vi "Begin.vi"(11 "Image Size":T1=enum."320x240") -> (0 "error out":errorcluster)   [LabVIEW 2012]
doc: "Called before other user functions, this VI is expected to open initial I/O refnums, load in file data, and do all program initialization. Notice that the <B>error out</B> terminal is simply used for data flow. Wiring it to other structures or subVIs ensures that this VI runs first."
uses:
  <vilib>/Rock Robotics/WPI/Camera/WPI_CameraImageSize.ctl
  <vilib>/Rock Robotics/WPI/Joystick/WPI_JoystickDeviceEnum.ctl
  <vilib>/Rock Robotics/WPI/Camera/WPI_CameraWhite Balance Values.ctl
  <vilib>/Rock Robotics/WPI/Camera/WPI_CameraExposure Values.ctl
  <vilib>/Rock Robotics/WPI/Camera/WPI_CameraFrameRate.ctl
  <vilib>/Rock Robotics/SystemInterfaces/Typedef/FPGA_TypedefDigitalModule.ctl
  <vilib>/Rock Robotics/SystemInterfaces/DIO/FPGA_DIOPWMChannel.ctl
  <vilib>/Rock Robotics/SystemInterfaces/DIO/FPGA_DIOChannel.ctl
  <vilib>/Rock Robotics/WPI/CAN/Jaguar/SubVIs/WPI_CANJaguar_SpeedReference.ctl
  <vilib>/Rock Robotics/WPI/CAN/Jaguar/SubVIs/WPI_CANJaguar_ControlMode.ctl
  <vilib>/Rock Robotics/WPI/CAN/Jaguar/SubVIs/WPI_CANJaguar_PositionReference.ctl
  <vilib>/Rock Robotics/SystemInterfaces/DIO/FPGA_DIORelayChannel.ctl
  <vilib>/Rock Robotics/WPI/Relay/WPI_RelayDirection.ctl
  <vilib>/Rock Robotics/WPI/MotorControl/WPI_MotorControlOpenCANJaguar.vi
  <vilib>/Rock Robotics/WPI/MotorControl/WPI_MotorControlOpen Victor.vi
  <vilib>/Rock Robotics/WPI/RobotDrive/WPI_RobotDriveOpen4MotorWithCANJaguar.vi
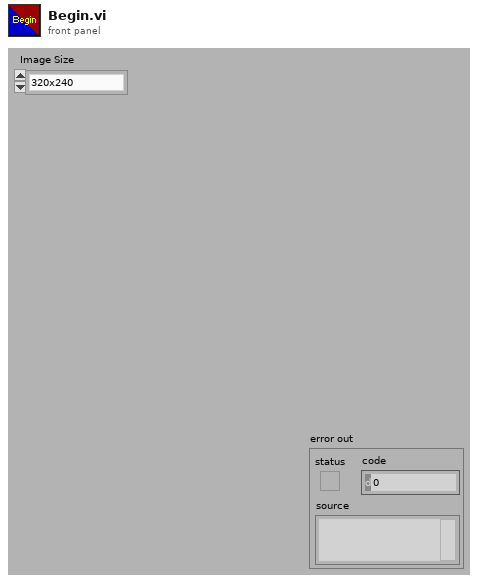
[diagram p1: front panel]
types:
  T1 = typedef "WPI_CameraImageSize.ctl" = enum16{"640x480", "320x240", "160x120"}
  T2 = typedef "WPI_CANJaguar_SpeedReference.ctl" = u8
  T3 = typedef "WPI_CANJaguar_ControlMode.ctl" = enum8{"Percent VBus", "Current", "Speed", "Position", "Voltage"}
  T4 = typedef "WPI_RelayDirection.ctl" = enum16{"Both directions", "Forward only", "Reverse only"}
  T5 = typedef "FPGA_DIORelayChannel.ctl" = enum8{"Relay 1", "Relay 2", "Relay 3", "Relay 4", "Relay 5", "Relay 6", "Relay 7", "Relay 8", "Invalid"}
  T6 = typedef "FPGA_DIOChannel.ctl" = enum8{"DIO 1", "DIO 2", "DIO 3", "DIO 4", "DIO 5", "DIO 6", "DIO 7", "DIO 8", "DIO 9", "DIO 10", "DIO 11", "DIO 12", "DIO 13", "DIO 14", "Invalid"}
  T7 = typedef "WPI_CANJaguar_PositionReference.ctl" = u8
  T8 = typedef "FPGA_DIOPWMChannel.ctl" = enum8{"PWM 1", "PWM 2", "PWM 3", "PWM 4", "PWM 5", "PWM 6", "PWM 7", "PWM 8", "PWM 9", "PWM 10", "Invalid"}
  T9 = typedef "FPGA_TypedefDigitalModule.ctl" = enum16{"Digital Module 1", "Digital Module 2"}
  T10 = typedef "WPI_JoystickDeviceEnum.ctl" = enum16{"USB 1", "USB 2", "USB 3", "USB 4", "Kinect 1", "Kinect 2"}
  T11 = typedef "WPI_CameraFrameRate.ctl" = u32
  T12 = typedef "WPI_CameraExposure Values.ctl" = enum16{"Auto", "Flicker-free 50 Hz", "Flicker-free 60 Hz", "Hold current"}
  T13 = typedef "WPI_CameraWhite Balance Values.ctl" = enum16{"Auto", "Fixed indoor", "Fixed outdoor 1", "Fixed outdoor 2", "Fixed fluorescent 1", "Fixed fluorescent 2", "Hold current"}
  T14 = typedef "WPI_RobotDriveDevRef.ctl" = cluster{"DevStatus":errorcluster, "Motors[]":T15[], "Square Inputs":bool, "Max Output":dbl, "Isochronous":bool}
  T15 = typedef "WPI_MotorControlDeviceRef.ctl" = cluster{"DeviceStatus":errorcluster, "Type":enum16{"PWM", "CAN"}, "PWM":cluster{"Digital Module":T9, "PWM Channel":T8, "DeadBand":T16}, "CAN":cluster{"Device Number":u8, "Control Mode":T3, "Semaphore":T17, "Max Vout":dbl}, "Invert":bool, "TransformRef":T18, "InvTransformRef":T18}
  T16 = typedef "WPI_PWMDeadband.ctl" = cluster{"Name":string, "maxPositivePwm":i32, "minPositivePwm":i32, "centerPwm":i32, "maxNegativePwm":i32, "minNegativePwm":i32, "angularRange":u16}
  T17 = typedef "Semaphore RefNum" = refnum<k1>
  T18 = typedef "WPI_PWMTransform_ConPane.ctl" = refnum<vi>
  T19 = typedef "WPI_JoystickDevRef.ctl" = cluster{"Device":T10}
  T20 = typedef "WPI_CameraDevRef.ctl" = cluster{"Camera Address":string, "CameraStatus":errorcluster, "Acquire Image Notifier":refnum<notifier>}
  T21 = typedef "WPI_DigitalInputDevRef.ctl" = cluster{"DevStatus":errorcluster, "DIO Channel":T6, "Digital Module":T9}
  T22 = typedef "WPI_RelayDevRef.ctl" = cluster{"DevStatus":errorcluster, "Relay Channel":T5, "Digital Module":T9, "Relay Direction":T4}
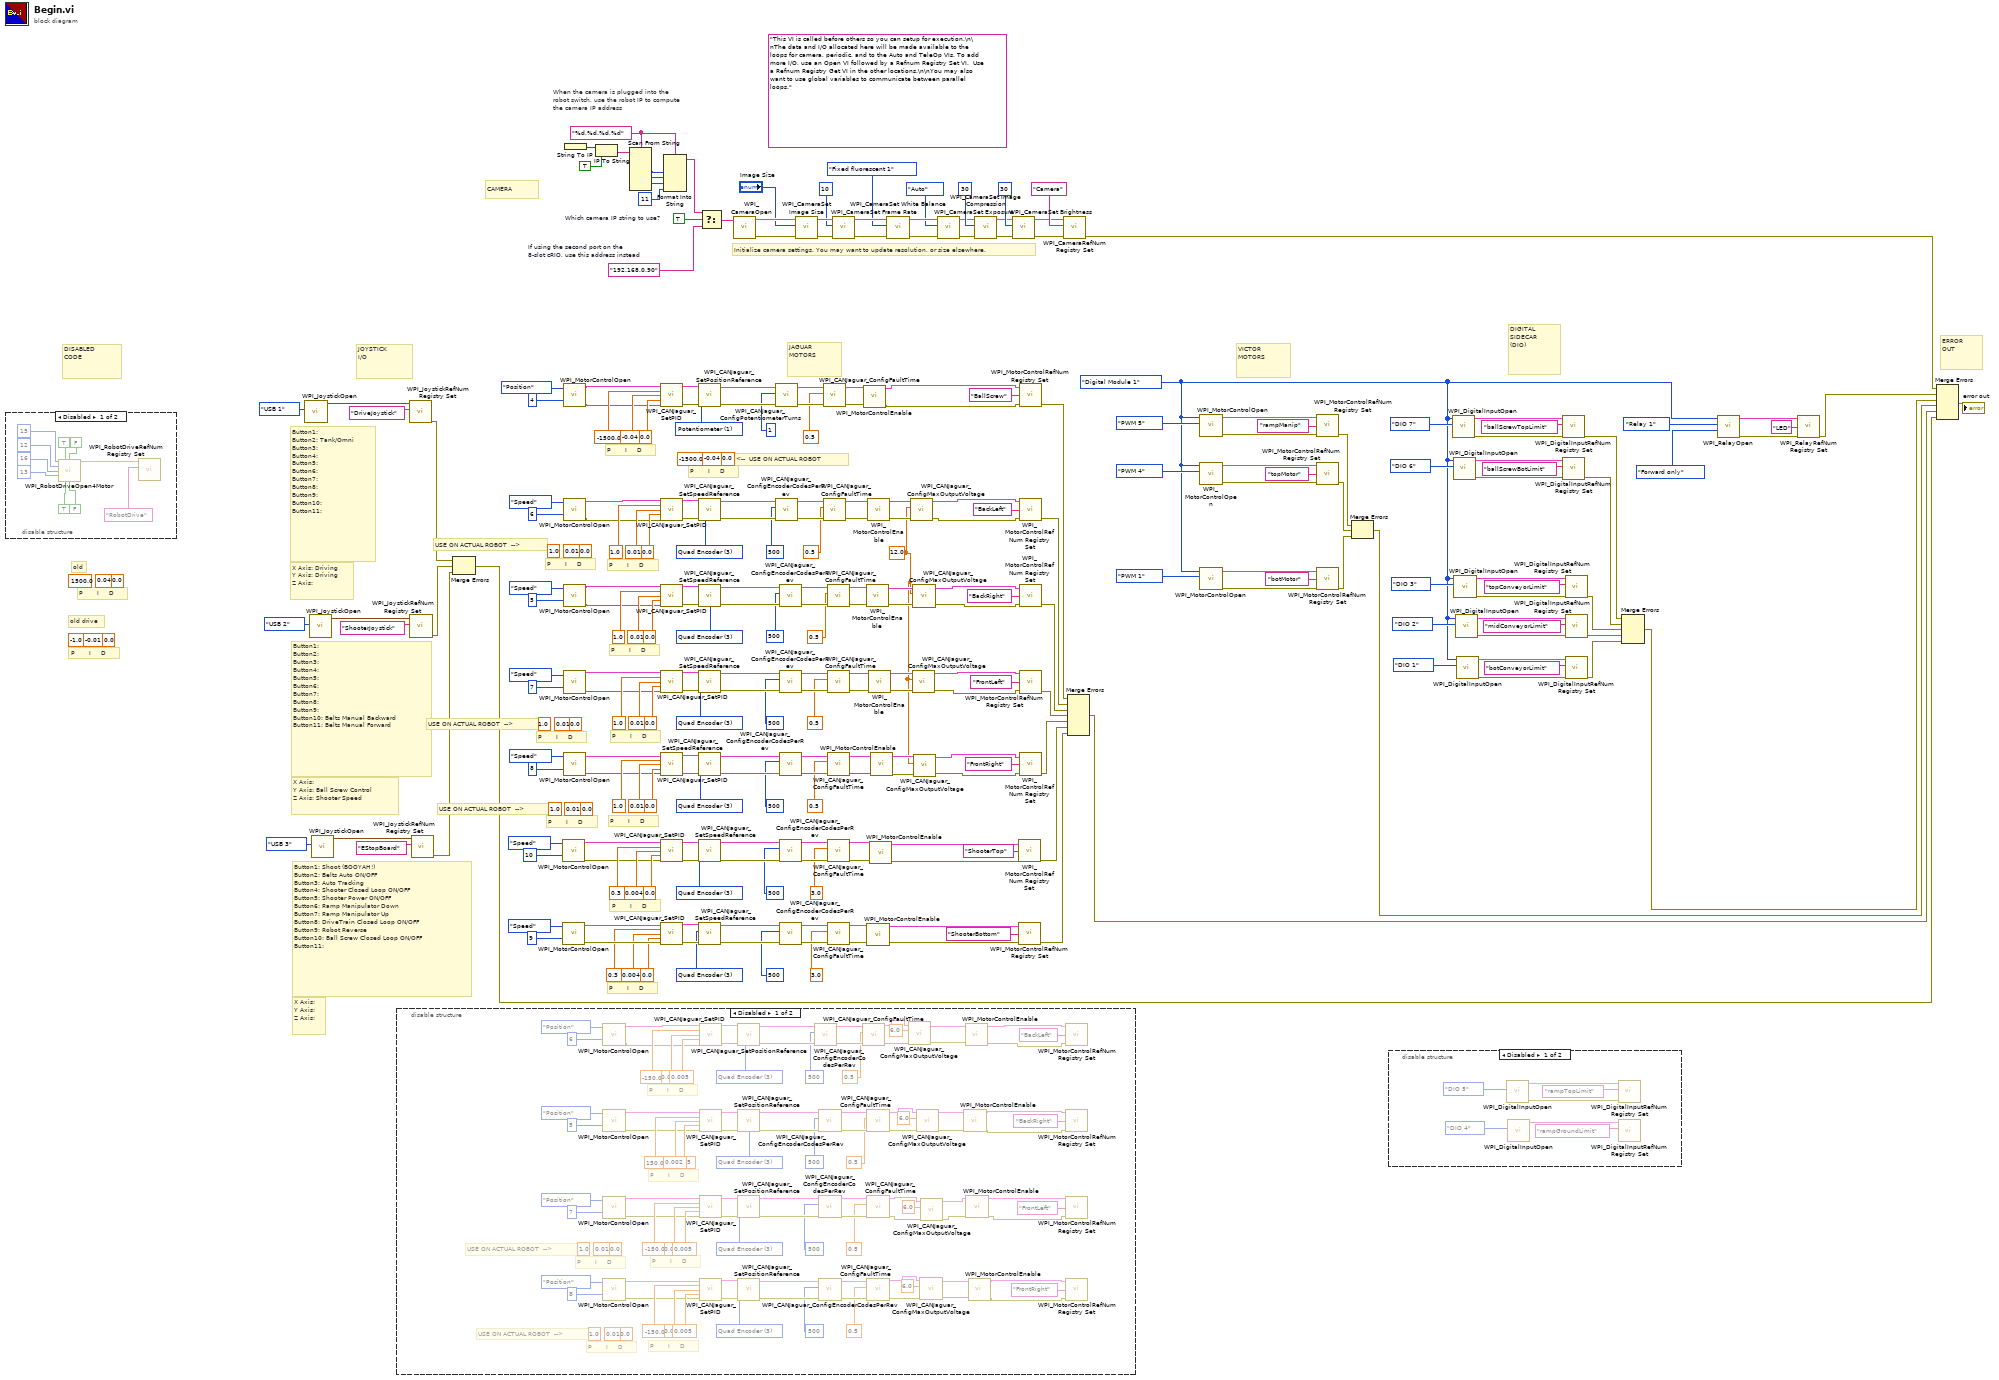
[diagram p0: block diagram]
diagram:
  (unwired) 0.0 ("D")
  (unwired) -0.01 ("I")
  (unwired) -1.0 ("P")
  (unwired) 0.0 ("D")
  (unwired) 0.04 ("I")
  (unwired) 1500.0 ("P")
  w4 = 12.0 ("Maximum Output Voltage")
  (unwired) 0.0 ("D")
  (unwired) 0.01 ("I")
  (unwired) 1.0 ("P")
  (unwired) 0.0 ("D")
  (unwired) 0.01 ("I")
  (unwired) 1.0 ("P")
  (unwired) 0.0 ("D")
  (unwired) 0.01 ("I")
  (unwired) 1.0 ("P")
  w37 = T2 3 items=["Encoder"=0, "Inv Encoder"=2, "Quad Encoder"=3, "None"=255] ("Speed Reference")
  w51 = T2 3 items=["Encoder"=0, "Inv Encoder"=2, "Quad Encoder"=3, "None"=255] ("Speed Reference")
  w65 = T2 3 items=["Encoder"=0, "Inv Encoder"=2, "Quad Encoder"=3, "None"=255] ("Speed Reference")
  w79 = T2 3 items=["Encoder"=0, "Inv Encoder"=2, "Quad Encoder"=3, "None"=255] ("Speed Reference")
  (unwired) 0.0 ("D")
  (unwired) -0.04 ("I")
  (unwired) -1500.0 ("P")
  w118 = T7 1 items=["Quad Encoder"=0, "Potentiometer"=1, "None"=255] ("Position Reference")
  w147 = T2 3 items=["Encoder"=0, "Inv Encoder"=2, "Quad Encoder"=3, "None"=255] ("Speed Reference")
  w161 = T2 3 items=["Encoder"=0, "Inv Encoder"=2, "Quad Encoder"=3, "None"=255] ("Speed Reference")
  w3 = FPGA_TypedefDigitalModule."Digital Module 1" ("Digital Module (Module 1)")
  w226 = TRUE  # Which camera IP string to use?
  w230 = "%d.%d.%d.%d" ("format string")
  (unwired) "This VI is called before others so you can setup for execution.\n\nThe data and I/O allocated here will be made available to the loops for camera, periodic, and to the Auto and TeleOp VIs. To add more I/O, use an Open VI followed by a Refnum Registry Set VI.  Use a Refnum Registry Get VI in the other locations.\n\nYou may also want to use global variables to communicate between parallel loops."
  w227 = "192.168.0.90"  # If using the second port on the 8-slot cRIO, use this address instead
  # "old drive"
  # "P       I     D"
  # "old"
  # "P       I     D"
  # "P       I     D"
  # "USE ON ACTUAL ROBOT  -->"
  # "P       I     D"
  # "USE ON ACTUAL ROBOT  -->"
  # "USE ON ACTUAL ROBOT  -->"
  # "P       I     D"
  # "P       I     D"
  # "P       I     D"
  # "P       I     D"
  # "P       I     D"
  # "<--  USE ON ACTUAL ROBOT"
  # "P       I     D"
  # "P       I     D"
  # "P       I     D"
  # "P       I     D"
  # "DIGITAL\nSIDECAR\n(DIO)"
  # "VICTOR\nMOTORS"
  # "X Axis:\nY Axis: \nZ Axis:"
  # "Button1: Shoot (BOOYAH!)\nButton2: Belts Auto ON/OFF\nButton3: Auto Tracking\nButton4: Shooter Closed Loop ON/OFF\nButton5: Shooter Power ON/OFF\nButton6: Ramp Manipulator Down\nButton7: Ramp Manipulator Up\nButton8: DriveTrain Closed Loop ON/OFF\nButton9: Robot Reverse\nButton10: Ball Screw Closed Loop ON/OFF\nButton11:"
  # "X Axis: \nY Axis: Ball Screw Control\nZ Axis: Shooter Speed"
  # "Button1:\nButton2: \nButton3:\nButton4:\nButton5:\nButton6:\nButton7:\nButton8:\nButton9:\nButton10: Belts Manual Backward\nButton11: Belts Manual Forward"
  # "X Axis: Driving\nY Axis: Driving\nZ Axis:"
  # "Button1:\nButton2: Tank/Omni\nButton3:\nButton4:\nButton5:\nButton6:\nButton7:\nButton8:\nButton9:\nButton10:\nButton11:"
  # "ERROR\nOUT"
  # "DISABLED\nCODE"
  # "CAMERA"
  # "JAGUAR\nMOTORS"
  # "JOYSTICK\nI/O"
  # "When the camera is plugged into the\nrobot switch, use the robot IP to compute\nthe camera IP address"
  # "Initialize camera settings. You may want to update resolution, or size elsewhere."
  n1 = disable-structure shown="Disabled" {
    frame Disabled {
      n2 = call-poly <vilib>:"WPI_RobotDriveOpen4Motor.vi"("Rear Left Motor"=u8 15, "Rear Left Motor Inverted"=TRUE, "Rear Right Motor Inverted"=FALSE, "Rear Right Motor"=u8 12, "Front Left Motor"=u8 16, "Front Right Motor"=u8 13, "Front Left Motor Inverted"=TRUE, "Front Right Motor Inverted"=FALSE) -> ("RobotDriveDevRef"=w263:T14)  [unwired: 6 in, 1 out]
      n3 = call <vilib>:"WPI_RobotDriveRefNum Registry Set.vi"("refnum name"="RobotDrive", "RobotDriveDevRef"=w263) -> ()  [unwired: 8 in, 2 out]
    }
    frame Enabled {
    }
  }
  n4 = call <vilib>:"WPI_JoystickOpen.vi"("JoystickDevice"=WPI_JoystickDeviceEnum."USB 1") -> ("JoystickDevRef"=w260:T19)  [unwired: 10 out]
  n5 = call <vilib>:"WPI_JoystickOpen.vi"("JoystickDevice"=WPI_JoystickDeviceEnum."USB 2") -> ("JoystickDevRef"=w211:T19)  [unwired: 10 out]
  n6 = call <vilib>:"WPI_JoystickOpen.vi"("JoystickDevice"=WPI_JoystickDeviceEnum."USB 3") -> ("JoystickDevRef"=w205:T19)  [unwired: 10 out]
  n7 = disable-structure shown="Disabled" {
    frame Disabled {
      (unwired) 0.0 ("D")
      (unwired) 0.01 ("I")
      (unwired) 1.0 ("P")
      (unwired) 0.0 ("D")
      (unwired) 0.01 ("I")
      (unwired) 1.0 ("P")
      w308 = T2 3 items=["Encoder"=0, "Inv Encoder"=2, "Quad Encoder"=3, "None"=255] ("Speed Reference")
      w322 = T2 3 items=["Encoder"=0, "Inv Encoder"=2, "Quad Encoder"=3, "None"=255] ("Speed Reference")
      w336 = T2 3 items=["Encoder"=0, "Inv Encoder"=2, "Quad Encoder"=3, "None"=255] ("Speed Reference")
      w350 = T2 3 items=["Encoder"=0, "Inv Encoder"=2, "Quad Encoder"=3, "None"=255] ("Speed Reference")
      # "P       I     D"
      # "USE ON ACTUAL ROBOT  -->"
      # "P       I     D"
      # "USE ON ACTUAL ROBOT  -->"
      # "P       I     D"
      # "P       I     D"
      # "P       I     D"
      # "P       I     D"
      n8 = call-poly <vilib>:"WPI_MotorControlOpen.vi"("Device Number"=u8 6, "Control Mode"=WPI_CANJaguar_ControlMode."Position") -> ("error out"=w300:errorcluster, "MotorControlDeviceRef"=w301:T15)  [unwired: 8 in]
      n9 = call-poly <vilib>:"WPI_MotorControlOpen.vi"("Device Number"=u8 5, "Control Mode"=WPI_CANJaguar_ControlMode."Position") -> ("error out"=w314:errorcluster, "MotorControlDeviceRef"=w315:T15)  [unwired: 8 in]
      n10 = call-poly <vilib>:"WPI_MotorControlOpen.vi"("Device Number"=u8 7, "Control Mode"=WPI_CANJaguar_ControlMode."Position") -> ("error out"=w328:errorcluster, "MotorControlDeviceRef"=w329:T15)  [unwired: 8 in]
      n11 = call-poly <vilib>:"WPI_MotorControlOpen.vi"("Device Number"=u8 8, "Control Mode"=WPI_CANJaguar_ControlMode."Position") -> ("error out"=w342:errorcluster, "MotorControlDeviceRef"=w343:T15)  [unwired: 8 in]
      n12 = call <vilib>:"WPI_CANJaguar_SetPID.vi"("CAN Jaguar Ref"=w301, "P"=-150.0, "I"=-0.002, "D"=0.005, "error in (no error)"=w300) -> ("CAN Jaguar Ref Out"=w309:T15, "error out"=w310:errorcluster)  [unwired: 9 in]
      n13 = call <vilib>:"WPI_CANJaguar_SetPID.vi"("CAN Jaguar Ref"=w315, "P"=150.0, "I"=0.002, "D"=0.005, "error in (no error)"=w314) -> ("CAN Jaguar Ref Out"=w323:T15, "error out"=w324:errorcluster)  [unwired: 9 in]
      n14 = call <vilib>:"WPI_CANJaguar_SetPID.vi"("CAN Jaguar Ref"=w329, "P"=-150.0, "I"=-0.002, "D"=0.005, "error in (no error)"=w328) -> ("CAN Jaguar Ref Out"=w337:T15, "error out"=w338:errorcluster)  [unwired: 9 in]
      n15 = call <vilib>:"WPI_CANJaguar_SetPID.vi"("CAN Jaguar Ref"=w343, "P"=-150.0, "I"=-0.002, "D"=0.005, "error in (no error)"=w342) -> ("CAN Jaguar Ref Out"=w351:T15, "error out"=w352:errorcluster)  [unwired: 9 in]
      n16 = call <vilib>:"WPI_CANJaguar_SetPositionReference.vi"("error in (no error)"=w310, "Position Reference"=w308, "CAN Jaguar Ref"=w309) -> ("error out"=w307:errorcluster, "CAN Jaguar Ref Out"=w306:T15)  [unwired: 7 in]
      n17 = call <vilib>:"WPI_CANJaguar_SetPositionReference.vi"("error in (no error)"=w324, "Position Reference"=w322, "CAN Jaguar Ref"=w323) -> ("error out"=w321:errorcluster, "CAN Jaguar Ref Out"=w320:T15)  [unwired: 7 in]
      n18 = call <vilib>:"WPI_CANJaguar_SetPositionReference.vi"("error in (no error)"=w338, "Position Reference"=w336, "CAN Jaguar Ref"=w337) -> ("error out"=w335:errorcluster, "CAN Jaguar Ref Out"=w334:T15)  [unwired: 7 in]
      n19 = call <vilib>:"WPI_CANJaguar_SetPositionReference.vi"("error in (no error)"=w352, "Position Reference"=w350, "CAN Jaguar Ref"=w351) -> ("error out"=w349:errorcluster, "CAN Jaguar Ref Out"=w348:T15)  [unwired: 7 in]
      n20 = call <vilib>:"WPI_CANJaguar_ConfigEncoderCodesPerRev.vi"("error in (no error)"=w307, "Encoder Codes Per Rev"=u16 500, "CAN Jaguar Ref"=w306) -> ("error out"=w304:errorcluster, "CAN Jaguar Ref Out"=w303:T15)  [unwired: 7 in]
      n21 = call <vilib>:"WPI_CANJaguar_ConfigEncoderCodesPerRev.vi"("error in (no error)"=w321, "Encoder Codes Per Rev"=u16 500, "CAN Jaguar Ref"=w320) -> ("error out"=w318:errorcluster, "CAN Jaguar Ref Out"=w317:T15)  [unwired: 7 in]
      n22 = call <vilib>:"WPI_CANJaguar_ConfigEncoderCodesPerRev.vi"("error in (no error)"=w335, "Encoder Codes Per Rev"=u16 500, "CAN Jaguar Ref"=w334) -> ("error out"=w332:errorcluster, "CAN Jaguar Ref Out"=w331:T15)  [unwired: 7 in]
      n23 = call <vilib>:"WPI_CANJaguar_ConfigEncoderCodesPerRev.vi"("error in (no error)"=w349, "Encoder Codes Per Rev"=u16 500, "CAN Jaguar Ref"=w348) -> ("error out"=w346:errorcluster, "CAN Jaguar Ref Out"=w345:T15)  [unwired: 7 in]
      n24 = call <vilib>:"WPI_CANJaguar_ConfigFaultTime.vi"("error in (no error)"=w304, "Fault Time (s)"=0.5, "CAN Jaguar Ref"=w303) -> ("error out"=w275:errorcluster, "CAN Jaguar Ref Out"=w272:T15)  [unwired: 7 in]
      n25 = call <vilib>:"WPI_CANJaguar_ConfigFaultTime.vi"("error in (no error)"=w318, "Fault Time (s)"=0.5, "CAN Jaguar Ref"=w317) -> ("error out"=w279:errorcluster, "CAN Jaguar Ref Out"=w276:T15)  [unwired: 7 in]
      n26 = call <vilib>:"WPI_CANJaguar_ConfigFaultTime.vi"("error in (no error)"=w332, "Fault Time (s)"=0.5, "CAN Jaguar Ref"=w331) -> ("error out"=w283:errorcluster, "CAN Jaguar Ref Out"=w280:T15)  [unwired: 7 in]
      n27 = call <vilib>:"WPI_CANJaguar_ConfigFaultTime.vi"("error in (no error)"=w346, "Fault Time (s)"=0.5, "CAN Jaguar Ref"=w345) -> ("error out"=w287:errorcluster, "CAN Jaguar Ref Out"=w284:T15)  [unwired: 7 in]
      n28 = call <vilib>:"WPI_CANJaguar_ConfigMaxOutputVoltage.vi"("error in (no error)"=w275, "Maximum Output Voltage"=6.0, "CAN Jaguar Ref"=w272) -> ("error out"=w274:errorcluster, "CAN Jaguar Ref Out"=w273:T15)  [unwired: 7 in]
      n29 = call <vilib>:"WPI_CANJaguar_ConfigMaxOutputVoltage.vi"("error in (no error)"=w279, "Maximum Output Voltage"=6.0, "CAN Jaguar Ref"=w276) -> ("error out"=w278:errorcluster, "CAN Jaguar Ref Out"=w277:T15)  [unwired: 7 in]
      n30 = call <vilib>:"WPI_CANJaguar_ConfigMaxOutputVoltage.vi"("error in (no error)"=w287, "Maximum Output Voltage"=6.0, "CAN Jaguar Ref"=w284) -> ("error out"=w286:errorcluster, "CAN Jaguar Ref Out"=w285:T15)  [unwired: 7 in]
      n31 = call <vilib>:"WPI_CANJaguar_ConfigMaxOutputVoltage.vi"("error in (no error)"=w283, "Maximum Output Voltage"=6.0, "CAN Jaguar Ref"=w280) -> ("error out"=w282:errorcluster, "CAN Jaguar Ref Out"=w281:T15)  [unwired: 7 in]
      n32 = call <vilib>:"WPI_MotorControlEnable.vi"("error in (no error)"=w278, "CAN Jaguar Ref"=w277) -> ("error out"=w296:errorcluster, "CAN Jaguar Ref Out"=w297:T15)  [unwired: 8 in]
      n33 = call <vilib>:"WPI_MotorControlEnable.vi"("error in (no error)"=w274, "CAN Jaguar Ref"=w273) -> ("error out"=w298:errorcluster, "CAN Jaguar Ref Out"=w299:T15)  [unwired: 8 in]
      n34 = call <vilib>:"WPI_MotorControlEnable.vi"("error in (no error)"=w282, "CAN Jaguar Ref"=w281) -> ("error out"=w295:errorcluster, "CAN Jaguar Ref Out"=w294:T15)  [unwired: 8 in]
      n35 = call <vilib>:"WPI_MotorControlEnable.vi"("error in (no error)"=w286, "CAN Jaguar Ref"=w285) -> ("error out"=w292:errorcluster, "CAN Jaguar Ref Out"=w293:T15)  [unwired: 8 in]
      n36 = call <vilib>:"WPI_MotorControlRefNum Registry Set.vi"("error in (no error)"=w298, "refnum name"="BackLeft", "MotorControlDevRef"=w299) -> ()  [unwired: 7 in, 2 out]
      n37 = call <vilib>:"WPI_MotorControlRefNum Registry Set.vi"("error in (no error)"=w296, "refnum name"="BackRight", "MotorControlDevRef"=w297) -> ()  [unwired: 7 in, 2 out]
      n38 = call <vilib>:"WPI_MotorControlRefNum Registry Set.vi"("error in (no error)"=w295, "refnum name"="FrontLeft", "MotorControlDevRef"=w294) -> ()  [unwired: 7 in, 2 out]
      n39 = call <vilib>:"WPI_MotorControlRefNum Registry Set.vi"("error in (no error)"=w292, "refnum name"="FrontRight", "MotorControlDevRef"=w293) -> ()  [unwired: 7 in, 2 out]
    }
    frame Enabled {
    }
  }
  n40 = call <vilib>:"WPI_JoystickRefNum Registry Set.vi"("refnum name"="DriveJoystick", "JoystickDevRef"=w260) -> ("error out"=w207:errorcluster)  [unwired: 1 in, 8 out]
  n41 = call <vilib>:"WPI_JoystickRefNum Registry Set.vi"("refnum name"="ShooterJoystick", "JoystickDevRef"=w211) -> ("error out"=w206:errorcluster)  [unwired: 1 in, 8 out]
  n42 = call <vilib>:"WPI_JoystickRefNum Registry Set.vi"("refnum name"="EStopBoard", "JoystickDevRef"=w205) -> ("error out"=w202:errorcluster)  [unwired: 1 in, 8 out]
  n43 = Merge Errors(w207, w206, w202) -> (w208:errorcluster)
  n44 = call-poly <vilib>:"WPI_MotorControlOpen.vi"("Device Number"=u8 10, "Control Mode"=WPI_CANJaguar_ControlMode."Speed") -> ("error out"=w137:errorcluster, "MotorControlDeviceRef"=w138:T15)  [unwired: 8 in]
  n45 = call-poly <vilib>:"WPI_MotorControlOpen.vi"("Device Number"=u8 9, "Control Mode"=WPI_CANJaguar_ControlMode."Speed") -> ("error out"=w167:errorcluster, "MotorControlDeviceRef"=w168:T15)  [unwired: 8 in]
  n46 = call-poly <vilib>:"WPI_MotorControlOpen.vi"("Device Number"=u8 4, "Control Mode"=WPI_CANJaguar_ControlMode."Position") -> ("error out"=w119:errorcluster, "MotorControlDeviceRef"=w120:T15)  [unwired: 8 in]
  n47 = call-poly <vilib>:"WPI_MotorControlOpen.vi"("Device Number"=u8 6, "Control Mode"=WPI_CANJaguar_ControlMode."Speed") -> ("error out"=w29:errorcluster, "MotorControlDeviceRef"=w30:T15)  [unwired: 8 in]
  n48 = call-poly <vilib>:"WPI_MotorControlOpen.vi"("Device Number"=u8 5, "Control Mode"=WPI_CANJaguar_ControlMode."Speed") -> ("error out"=w43:errorcluster, "MotorControlDeviceRef"=w44:T15)  [unwired: 8 in]
  n49 = call-poly <vilib>:"WPI_MotorControlOpen.vi"("Device Number"=u8 7, "Control Mode"=WPI_CANJaguar_ControlMode."Speed") -> ("error out"=w57:errorcluster, "MotorControlDeviceRef"=w58:T15)  [unwired: 8 in]
  n50 = call-poly <vilib>:"WPI_MotorControlOpen.vi"("Device Number"=u8 8, "Control Mode"=WPI_CANJaguar_ControlMode."Speed") -> ("error out"=w71:errorcluster, "MotorControlDeviceRef"=w72:T15)  [unwired: 8 in]
  n51 = String To IP() -> (0:w237:u32)  [unwired: 1 in]
  n52 = IP To String(1:TRUE ("dot notation? (F)"), 2:w237) -> (0:w235:string)
  n53 = Scan From String(format string=w230, input string=w235) -> (output 1=w234:i32, output 2=w233:i32, output 3=w232:i32)  [unwired: 7 in, 3 out]
  n54 = call <vilib>:"WPI_CANJaguar_SetPID.vi"("CAN Jaguar Ref"=w120, "P"=-1500.0, "I"=-0.04, "D"=0.0, "error in (no error)"=w119) -> ("CAN Jaguar Ref Out"=w126:T15, "error out"=w127:errorcluster)  [unwired: 9 in]
  n55 = call <vilib>:"WPI_CANJaguar_SetPID.vi"("CAN Jaguar Ref"=w30, "P"=1.0, "I"=0.01, "D"=0.0, "error in (no error)"=w29) -> ("CAN Jaguar Ref Out"=w38:T15, "error out"=w39:errorcluster)  [unwired: 9 in]
  n56 = call <vilib>:"WPI_CANJaguar_SetPID.vi"("CAN Jaguar Ref"=w44, "P"=1.0, "I"=0.01, "D"=0.0, "error in (no error)"=w43) -> ("CAN Jaguar Ref Out"=w52:T15, "error out"=w53:errorcluster)  [unwired: 9 in]
  n57 = call <vilib>:"WPI_CANJaguar_SetPID.vi"("CAN Jaguar Ref"=w58, "P"=1.0, "I"=0.01, "D"=0.0, "error in (no error)"=w57) -> ("CAN Jaguar Ref Out"=w66:T15, "error out"=w67:errorcluster)  [unwired: 9 in]
  n58 = call <vilib>:"WPI_CANJaguar_SetPID.vi"("CAN Jaguar Ref"=w72, "P"=1.0, "I"=0.01, "D"=0.0, "error in (no error)"=w71) -> ("CAN Jaguar Ref Out"=w80:T15, "error out"=w81:errorcluster)  [unwired: 9 in]
  n59 = call <vilib>:"WPI_CANJaguar_SetPID.vi"("CAN Jaguar Ref"=w138, "P"=0.3, "I"=0.004, "D"=0.0, "error in (no error)"=w137) -> ("CAN Jaguar Ref Out"=w148:T15, "error out"=w149:errorcluster)  [unwired: 9 in]
  n60 = call <vilib>:"WPI_CANJaguar_SetPID.vi"("CAN Jaguar Ref"=w168, "P"=0.3, "I"=0.004, "D"=0.0, "error in (no error)"=w167) -> ("CAN Jaguar Ref Out"=w162:T15, "error out"=w163:errorcluster)  [unwired: 9 in]
  n61 = Format Into String(format string=w230, w234, w233, w232, 11 ("Compression")) -> (resulting string=w228:string)  [unwired: 2 in, 1 out]
  n62 = call <vilib>:"WPI_CANJaguar_SetPositionReference.vi"("error in (no error)"=w127, "Position Reference"=w118, "CAN Jaguar Ref"=w126) -> ("error out"=w125:errorcluster, "CAN Jaguar Ref Out"=w124:T15)  [unwired: 7 in]
  n63 = call <vilib>:"WPI_CANJaguar_SetSpeedReference.vi"("error in (no error)"=w39, "Speed Reference"=w37, "CAN Jaguar Ref"=w38) -> ("error out"=w36:errorcluster, "CAN Jaguar Ref Out"=w35:T15)  [unwired: 7 in]
  n64 = call <vilib>:"WPI_CANJaguar_SetSpeedReference.vi"("error in (no error)"=w53, "Speed Reference"=w51, "CAN Jaguar Ref"=w52) -> ("error out"=w50:errorcluster, "CAN Jaguar Ref Out"=w49:T15)  [unwired: 7 in]
  n65 = call <vilib>:"WPI_CANJaguar_SetSpeedReference.vi"("error in (no error)"=w67, "Speed Reference"=w65, "CAN Jaguar Ref"=w66) -> ("error out"=w64:errorcluster, "CAN Jaguar Ref Out"=w63:T15)  [unwired: 7 in]
  n66 = call <vilib>:"WPI_CANJaguar_SetSpeedReference.vi"("error in (no error)"=w81, "Speed Reference"=w79, "CAN Jaguar Ref"=w80) -> ("error out"=w78:errorcluster, "CAN Jaguar Ref Out"=w77:T15)  [unwired: 7 in]
  n67 = call <vilib>:"WPI_CANJaguar_SetSpeedReference.vi"("error in (no error)"=w149, "Speed Reference"=w147, "CAN Jaguar Ref"=w148) -> ("error out"=w146:errorcluster, "CAN Jaguar Ref Out"=w145:T15)  [unwired: 7 in]
  n68 = call <vilib>:"WPI_CANJaguar_SetSpeedReference.vi"("error in (no error)"=w163, "Speed Reference"=w161, "CAN Jaguar Ref"=w162) -> ("error out"=w160:errorcluster, "CAN Jaguar Ref Out"=w159:T15)  [unwired: 7 in]
  n69 = Select(t=w228, s=w226, f=w227) -> (s? t:f=w229:string)
  n70 = call <vilib>:"WPI_CameraOpen.vi"("Camera Address"=w229) -> ("error out"=w250:errorcluster, "CameraDevRef"=w251:T20)  [unwired: 1 in, 8 out]
  n71 = call <vilib>:"WPI_CANJaguar_ConfigPotentiometerTurns.vi"("error in (no error)"=w125, "Potentiometer Turns"=u16 1, "CAN Jaguar Ref"=w124) -> ("error out"=w123:errorcluster, "CAN Jaguar Ref Out"=w122:T15)  [unwired: 7 in]
  n72 = call <vilib>:"WPI_CANJaguar_ConfigEncoderCodesPerRev.vi"("error in (no error)"=w36, "Encoder Codes Per Rev"=u16 500, "CAN Jaguar Ref"=w35) -> ("error out"=w33:errorcluster, "CAN Jaguar Ref Out"=w32:T15)  [unwired: 7 in]
  n73 = call <vilib>:"WPI_CANJaguar_ConfigEncoderCodesPerRev.vi"("error in (no error)"=w50, "Encoder Codes Per Rev"=u16 500, "CAN Jaguar Ref"=w49) -> ("error out"=w47:errorcluster, "CAN Jaguar Ref Out"=w46:T15)  [unwired: 7 in]
  n74 = call <vilib>:"WPI_CANJaguar_ConfigEncoderCodesPerRev.vi"("error in (no error)"=w64, "Encoder Codes Per Rev"=u16 500, "CAN Jaguar Ref"=w63) -> ("error out"=w61:errorcluster, "CAN Jaguar Ref Out"=w60:T15)  [unwired: 7 in]
  n75 = call <vilib>:"WPI_CANJaguar_ConfigEncoderCodesPerRev.vi"("error in (no error)"=w78, "Encoder Codes Per Rev"=u16 500, "CAN Jaguar Ref"=w77) -> ("error out"=w75:errorcluster, "CAN Jaguar Ref Out"=w74:T15)  [unwired: 7 in]
  n76 = call <vilib>:"WPI_CANJaguar_ConfigEncoderCodesPerRev.vi"("error in (no error)"=w146, "Encoder Codes Per Rev"=u16 500, "CAN Jaguar Ref"=w145) -> ("error out"=w143:errorcluster, "CAN Jaguar Ref Out"=w142:T15)  [unwired: 7 in]
  n77 = call <vilib>:"WPI_CANJaguar_ConfigEncoderCodesPerRev.vi"("error in (no error)"=w160, "Encoder Codes Per Rev"=u16 500, "CAN Jaguar Ref"=w159) -> ("error out"=w157:errorcluster, "CAN Jaguar Ref Out"=w156:T15)  [unwired: 7 in]
  n78 = call <vilib>:"WPI_CameraSet Image Size.vi"("error in (no error)"=w250, "Image Size"="Image Size", "CameraDevRef"=w251) -> ("error out"=w249:errorcluster, "CameraDevRef Out"=w252:T20)  [unwired: 7 out]
  n79 = call <vilib>:"WPI_CANJaguar_ConfigFaultTime.vi"("error in (no error)"=w123, "Fault Time (s)"=0.5, "CAN Jaguar Ref"=w122) -> ("error out"=w107:errorcluster, "CAN Jaguar Ref Out"=w108:T15)  [unwired: 7 in]
  n80 = call <vilib>:"WPI_CANJaguar_ConfigFaultTime.vi"("error in (no error)"=w33, "Fault Time (s)"=0.5, "CAN Jaguar Ref"=w32) -> ("error out"=w28:errorcluster, "CAN Jaguar Ref Out"=w27:T15)  [unwired: 7 in]
  n81 = call <vilib>:"WPI_CANJaguar_ConfigFaultTime.vi"("error in (no error)"=w47, "Fault Time (s)"=0.5, "CAN Jaguar Ref"=w46) -> ("error out"=w25:errorcluster, "CAN Jaguar Ref Out"=w26:T15)  [unwired: 7 in]
  n82 = call <vilib>:"WPI_CANJaguar_ConfigFaultTime.vi"("error in (no error)"=w61, "Fault Time (s)"=0.5, "CAN Jaguar Ref"=w60) -> ("error out"=w23:errorcluster, "CAN Jaguar Ref Out"=w24:T15)  [unwired: 7 in]
  n83 = call <vilib>:"WPI_CANJaguar_ConfigFaultTime.vi"("error in (no error)"=w75, "Fault Time (s)"=0.5, "CAN Jaguar Ref"=w74) -> ("error out"=w22:errorcluster, "CAN Jaguar Ref Out"=w21:T15)  [unwired: 7 in]
  n84 = call <vilib>:"WPI_CANJaguar_ConfigFaultTime.vi"("error in (no error)"=w143, "Fault Time (s)"=3.0, "CAN Jaguar Ref"=w142) -> ("error out"=w139:errorcluster, "CAN Jaguar Ref Out"=w140:T15)  [unwired: 7 in]
  n85 = call <vilib>:"WPI_CANJaguar_ConfigFaultTime.vi"("error in (no error)"=w157, "Fault Time (s)"=3.0, "CAN Jaguar Ref"=w156) -> ("error out"=w153:errorcluster, "CAN Jaguar Ref Out"=w154:T15)  [unwired: 7 in]
  n86 = call <vilib>:"WPI_CameraSet Frame Rate.vi"("error in (no error)"=w249, "Frame Rate (fps)"=T11 10, "CameraDevRef"=w252) -> ("error out"=w248:errorcluster, "CameraDevRef Out"=w254:T20)  [unwired: 7 out]
  n87 = call <vilib>:"WPI_MotorControlEnable.vi"("error in (no error)"=w107, "CAN Jaguar Ref"=w108) -> ("error out"=w106:errorcluster, "CAN Jaguar Ref Out"=w105:T15)  [unwired: 8 in]
  n88 = call <vilib>:"WPI_MotorControlEnable.vi"("error in (no error)"=w25, "CAN Jaguar Ref"=w26) -> ("error out"=w16:errorcluster, "CAN Jaguar Ref Out"=w15:T15)  [unwired: 8 in]
  n89 = call <vilib>:"WPI_MotorControlEnable.vi"("error in (no error)"=w153, "CAN Jaguar Ref"=w154) -> ("error out"=w169:errorcluster, "CAN Jaguar Ref Out"=w170:T15)  [unwired: 8 in]
  n90 = call <vilib>:"WPI_MotorControlEnable.vi"("error in (no error)"=w28, "CAN Jaguar Ref"=w27) -> ("error out"=w19:errorcluster, "CAN Jaguar Ref Out"=w20:T15)  [unwired: 8 in]
  n91 = call <vilib>:"WPI_MotorControlEnable.vi"("error in (no error)"=w23, "CAN Jaguar Ref"=w24) -> ("error out"=w11:errorcluster, "CAN Jaguar Ref Out"=w12:T15)  [unwired: 8 in]
  n92 = call <vilib>:"WPI_MotorControlEnable.vi"("error in (no error)"=w139, "CAN Jaguar Ref"=w140) -> ("error out"=w136:errorcluster, "CAN Jaguar Ref Out"=w135:T15)  [unwired: 8 in]
  n93 = call <vilib>:"WPI_MotorControlEnable.vi"("error in (no error)"=w22, "CAN Jaguar Ref"=w21) -> ("error out"=w5:errorcluster, "CAN Jaguar Ref Out"=w8:T15)  [unwired: 8 in]
  n94 = call <vilib>:"WPI_CameraSet White Balance.vi"("error in (no error)"=w248, "White Balance"=WPI_CameraWhite_Balance_Values."Fixed fluorescent 1", "CameraDevRef"=w254) -> ("error out"=w247:errorcluster, "CameraDevRef Out"=w253:T20)  [unwired: 7 out]
  n95 = call <vilib>:"WPI_CANJaguar_ConfigMaxOutputVoltage.vi"("error in (no error)"=w19, "Maximum Output Voltage"=w4, "CAN Jaguar Ref"=w20) -> ("error out"=w18:errorcluster, "CAN Jaguar Ref Out"=w17:T15)  [unwired: 7 in]
  n96 = call <vilib>:"WPI_CANJaguar_ConfigMaxOutputVoltage.vi"("error in (no error)"=w11, "Maximum Output Voltage"=w4, "CAN Jaguar Ref"=w12) -> ("error out"=w10:errorcluster, "CAN Jaguar Ref Out"=w9:T15)  [unwired: 7 in]
  n97 = call <vilib>:"WPI_CANJaguar_ConfigMaxOutputVoltage.vi"("error in (no error)"=w16, "Maximum Output Voltage"=w4, "CAN Jaguar Ref"=w15) -> ("error out"=w13:errorcluster, "CAN Jaguar Ref Out"=w14:T15)  [unwired: 7 in]
  n98 = call <vilib>:"WPI_CANJaguar_ConfigMaxOutputVoltage.vi"("error in (no error)"=w5, "Maximum Output Voltage"=w4, "CAN Jaguar Ref"=w8) -> ("error out"=w6:errorcluster, "CAN Jaguar Ref Out"=w7:T15)  [unwired: 7 in]
  n99 = call <vilib>:"WPI_CameraSet Exposure.vi"("error in (no error)"=w247, "Exposure"=WPI_CameraExposure_Values."Auto", "CameraDevRef"=w253) -> ("error out"=w246:errorcluster, "CameraDevRef Out"=w256:T20)  [unwired: 7 out]
  n100 = call <vilib>:"WPI_CameraSet Image Compression.vi"("error in (no error)"=w246, "Compression"=30, "CameraDevRef"=w256) -> ("error out"=w245:errorcluster, "CameraDevRef Out"=w255:T20)  [unwired: 7 out]
  n101 = call <vilib>:"WPI_CameraSet Brightness.vi"("error in (no error)"=w245, "Brightness"=30, "CameraDevRef"=w255) -> ("error out"=w243:errorcluster, "CameraDevRef Out"=w244:T20)  [unwired: 7 out]
  n102 = call <vilib>:"WPI_MotorControlRefNum Registry Set.vi"("error in (no error)"=w136, "refnum name"="ShooterTop", "MotorControlDevRef"=w135) -> ("error out"=w213:errorcluster)  [unwired: 7 in, 1 out]
  n103 = call <vilib>:"WPI_MotorControlRefNum Registry Set.vi"("error in (no error)"=w169, "refnum name"="ShooterBottom", "MotorControlDevRef"=w170) -> ("error out"=w212:errorcluster)  [unwired: 7 in, 1 out]
  n104 = call <vilib>:"WPI_MotorControlRefNum Registry Set.vi"("error in (no error)"=w106, "refnum name"="BallScrew", "MotorControlDevRef"=w105) -> ("error out"=w131:errorcluster)  [unwired: 7 in, 1 out]
  n105 = call <vilib>:"WPI_MotorControlRefNum Registry Set.vi"("error in (no error)"=w18, "refnum name"="BackLeft", "MotorControlDevRef"=w17) -> ("error out"=w224:errorcluster)  [unwired: 7 in, 1 out]
  n106 = call <vilib>:"WPI_MotorControlRefNum Registry Set.vi"("error in (no error)"=w13, "refnum name"="BackRight", "MotorControlDevRef"=w14) -> ("error out"=w223:errorcluster)  [unwired: 7 in, 1 out]
  n107 = call <vilib>:"WPI_MotorControlRefNum Registry Set.vi"("error in (no error)"=w10, "refnum name"="FrontLeft", "MotorControlDevRef"=w9) -> ("error out"=w222:errorcluster)  [unwired: 7 in, 1 out]
  n108 = call <vilib>:"WPI_MotorControlRefNum Registry Set.vi"("error in (no error)"=w6, "refnum name"="FrontRight", "MotorControlDevRef"=w7) -> ("error out"=w221:errorcluster)  [unwired: 7 in, 1 out]
  n109 = call <vilib>:"WPI_CameraRefNum Registry Set.vi"("error in (no error)"=w243, "refnum name"="Camera", "CameraDevRef"=w244) -> ("error out"=w98:errorcluster)  [unwired: 8 out]
  n110 = Merge Errors(w131, w224, w223, w222, w221, w213, w212) -> (w220:errorcluster)
  n111 = call-poly <vilib>:"WPI_MotorControlOpen.vi"("PWM Channel"=FPGA_DIOPWMChannel."PWM 5", "Digital Module (Module 1)"=w3) -> ("error out"=w175:errorcluster, "MotorControlDeviceRef"=w174:T15)  [unwired: 8 in]
  n112 = call-poly <vilib>:"WPI_MotorControlOpen.vi"("PWM Channel"=FPGA_DIOPWMChannel."PWM 4", "Digital Module (Module 1)"=w3) -> ("error out"=w201:errorcluster, "MotorControlDeviceRef"=w200:T15)  [unwired: 8 in]
  n113 = call-poly <vilib>:"WPI_MotorControlOpen.vi"("PWM Channel"=FPGA_DIOPWMChannel."PWM 1", "Digital Module (Module 1)"=w3) -> ("error out"=w198:errorcluster, "MotorControlDeviceRef"=w197:T15)  [unwired: 8 in]
  n114 = call <vilib>:"WPI_MotorControlRefNum Registry Set.vi"("error in (no error)"=w175, "refnum name"="rampManip", "MotorControlDevRef"=w174) -> ("error out"=w171:errorcluster)  [unwired: 7 in, 1 out]
  n115 = call <vilib>:"WPI_MotorControlRefNum Registry Set.vi"("error in (no error)"=w201, "refnum name"="topMotor", "MotorControlDevRef"=w200) -> ("error out"=w193:errorcluster)  [unwired: 7 in, 1 out]
  n116 = call <vilib>:"WPI_MotorControlRefNum Registry Set.vi"("error in (no error)"=w198, "refnum name"="botMotor", "MotorControlDevRef"=w197) -> ("error out"=w104:errorcluster)  [unwired: 7 in, 1 out]
  n117 = Merge Errors(w171, w193, w104) -> (w192:errorcluster)
  n118 = disable-structure shown="Disabled" {
    frame Disabled {
      n119 = call <vilib>:"WPI_DigitalInputOpen.vi"("DIO Channel"=FPGA_DIOChannel."DIO 5") -> ("error out"=w373:errorcluster, "DigitalInputDevRef"=w374:T21)  [unwired: 9 in]
      n120 = call <vilib>:"WPI_DigitalInputOpen.vi"("DIO Channel"=FPGA_DIOChannel."DIO 4") -> ("DigitalInputDevRef"=w368:T21)  [unwired: 9 in, 1 out]
      n121 = call <vilib>:"WPI_DigitalInputRefNum Registry Set.vi"("error in (no error)"=w373, "refnum name"="rampTopLimit", "DigitalInputDevRef"=w374) -> ()  [unwired: 7 in, 2 out]
      n122 = call <vilib>:"WPI_DigitalInputRefNum Registry Set.vi"("refnum name"="rampGroundLimit", "DigitalInputDevRef"=w368) -> ()  [unwired: 8 in, 2 out]
    }
    frame Enabled {
    }
  }
  n123 = call <vilib>:"WPI_DigitalInputOpen.vi"("DIO Channel"=FPGA_DIOChannel."DIO 7", "Digital Module (Module 1)"=w3) -> ("error out"=w116:errorcluster, "DigitalInputDevRef"=w113:T21)  [unwired: 8 in]
  n124 = call <vilib>:"WPI_DigitalInputOpen.vi"("DIO Channel"=FPGA_DIOChannel."DIO 6", "Digital Module (Module 1)"=w3) -> ("error out"=w112:errorcluster, "DigitalInputDevRef"=w109:T21)  [unwired: 8 in]
  n125 = call <vilib>:"WPI_DigitalInputOpen.vi"("DIO Channel"=FPGA_DIOChannel."DIO 3", "Digital Module (Module 1)"=w3) -> ("error out"=w190:errorcluster, "DigitalInputDevRef"=w191:T21)  [unwired: 8 in]
  n126 = call <vilib>:"WPI_DigitalInputOpen.vi"("DIO Channel"=FPGA_DIOChannel."DIO 2", "Digital Module (Module 1)"=w3) -> ("error out"=w187:errorcluster, "DigitalInputDevRef"=w184:T21)  [unwired: 8 in]
  n127 = call <vilib>:"WPI_DigitalInputOpen.vi"("DIO Channel"=FPGA_DIOChannel."DIO 1", "Digital Module (Module 1)"=w3) -> ("error out"=w183:errorcluster, "DigitalInputDevRef"=w180:T21)  [unwired: 8 in]
  n128 = call <vilib>:"WPI_DigitalInputRefNum Registry Set.vi"("error in (no error)"=w116, "refnum name"="ballScrewTopLimit", "DigitalInputDevRef"=w113) -> ("error out"=w1:errorcluster)  [unwired: 7 in, 1 out]
  n129 = call <vilib>:"WPI_DigitalInputRefNum Registry Set.vi"("error in (no error)"=w112, "refnum name"="ballScrewBotLimit", "DigitalInputDevRef"=w109) -> ("error out"=w2:errorcluster)  [unwired: 7 in, 1 out]
  n130 = call <vilib>:"WPI_DigitalInputRefNum Registry Set.vi"("error in (no error)"=w190, "refnum name"="topConveyorLimit", "DigitalInputDevRef"=w191) -> ("error out"=w178:errorcluster)  [unwired: 7 in, 1 out]
  n131 = call <vilib>:"WPI_DigitalInputRefNum Registry Set.vi"("error in (no error)"=w187, "refnum name"="midConveyorLimit", "DigitalInputDevRef"=w184) -> ("error out"=w179:errorcluster)  [unwired: 7 in, 1 out]
  n132 = call <vilib>:"WPI_DigitalInputRefNum Registry Set.vi"("error in (no error)"=w183, "refnum name"="botConveyorLimit", "DigitalInputDevRef"=w180) -> ("error out"=w177:errorcluster)  [unwired: 7 in, 1 out]
  n133 = Merge Errors(w1, w2, w178, w179, w177) -> (w176:errorcluster)
  n134 = call <vilib>:"WPI_RelayOpen.vi"("Relay Direction"=WPI_RelayDirection."Forward only", "Relay Channel"=FPGA_DIORelayChannel."Relay 1", "Digital Module (Module 1)"=w3) -> ("error out"=w102:errorcluster, "RelayDevRef"=w103:T22)  [unwired: 7 in]
  n135 = call <vilib>:"WPI_RelayRefNum Registry Set.vi"("error in (no error)"=w102, "refnum name"="LED", "RelayDevRef"=w103) -> ("error out"=w97:errorcluster)  [unwired: 7 in, 1 out]
  n136 = Merge Errors(w98, w97, w176, w192, w220, w208) -> (→"error out":errorcluster)
